vi "FT10_Connect Hardware.vi"(0 "Message Handling Cluster in":T1, 11 "error in (no error)":errorcluster) -> (4 "Message Handling Cluster out":T1, 6 "Fornax Connected?":bool, 8 "Unitherm Connected?":bool, 10 "M4X Connected?":bool, 14 "PXI-7854R Connected?":bool, 15 "error out":errorcluster)   [LabVIEW 2024]
doc: "Connects to Fornax, Unitherm, and M4X. Then bundles connections into cluster."
uses:
  Controls/Control_Message Handling Cluster.ctl
  Controls/Control_M4X Connection.ctl
  Controls/Control_PXI-7854R FPGA Reference.ctl
  <vilib>/userDefined/High Color/nirio_resource_hc.ctl
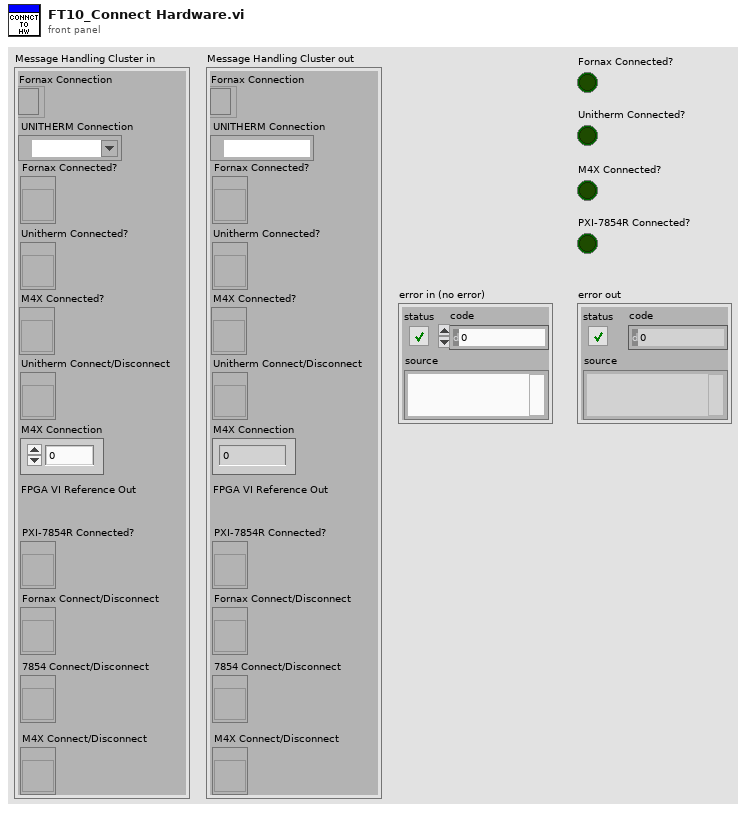
[diagram p1: front panel]
types:
  T1 = typedef "Control_Message Handling Cluster.ctl" = cluster{"Fornax Connected?":refnum<vi>, "Unitherm Connected?":refnum<vi>, "M4X Connected?":refnum<vi>, "Unitherm Connect/Disconnect":refnum<vi>, "Fornax Connection":refnum<k5>, "UNITHERM Connection":refnum<visa-resource-name>, "M4X Connection":T2, "PXI-7854R FPGA Reference":T3, "PXI-7854R Connected?":refnum<vi>, "Fornax Connect/Disconnect":refnum<vi>, "7854 Connect/Disconnect":refnum<vi>, "M4X Connect/Disconnect":refnum<vi>}
  T2 = typedef "Control_M4X Connection.ctl" = u32
  T3 = typedef "Control_PXI-7854R FPGA Reference.ctl" = refnum<k20>
  T4 = typedef "nirio_resource_hc.ctl" = tag
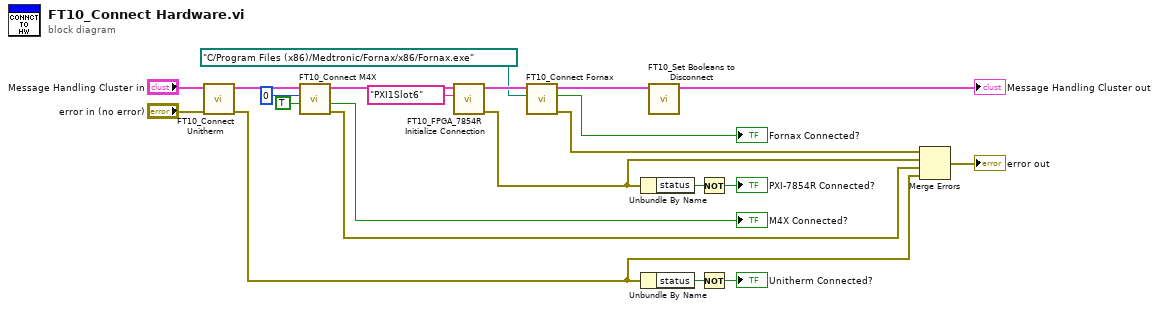
[diagram p0: block diagram]
diagram:
  n1 = call "FT10_Connect Unitherm.vi"("error in (no error)"="error in (no error)", "Message Handling Cluster in"="Message Handling Cluster in") -> ("error out"=w5:errorcluster, "Message Handling Cluster out"=w4:T1)  [unwired: 8 in]
  n2 = call "FT10_Connect M4X.vi"("reset device"=TRUE, "Board #"=u32 0, "Message Handling Cluster in"=w4) -> ("error out"=w12:errorcluster, "M4X Connected?"=→"M4X Connected?":bool, "Message Handling Cluster out"=w13:T1)  [unwired: 5 in, 1 out]
  n3 = call "FT10_FPGA_7854R Initialize Connection.vi"("FPGA resource name"=T4 "PXI1Slot6", "Message Handling Cluster in"=w13) -> ("error out"=w11:errorcluster, "Message Handling Cluster out"=w8:T1)  [unwired: 7 in, 1 out]
  n4 = call "FT10_Connect Fornax.vi"("Fornax Executable Path"=path "C:/Program Files (x86)/Medtronic/Fornax/x86/Fornax.exe", "Message Handling Cluster in"=w8) -> ("error out"=w20:errorcluster, "Fornax Connected?"=→"Fornax Connected?":bool, "Message Handling Cluster out"=w3:T1)  [unwired: 7 in]
  n5 = Unbundle By Name(w11) -> ("status"=w10:bool)
  n6 = Unbundle By Name(w5) -> ("status"=w21:bool)
  n7 = call "FT10_Set Booleans to Disconnect.vi"("Message Handling Cluster in"=w3) -> ("Message Handling Cluster out"=→"Message Handling Cluster out":T1)  [unwired: 10 in]
  n8 = Not(x=w10) -> (.not. x?=→"PXI-7854R Connected?":bool)
  n9 = Not(x=w21) -> (.not. x?=→"Unitherm Connected?":bool)
  n10 = Merge Errors(w20, w11, w12, w5) -> (→"error out":errorcluster)
